vi "Main.vi"() -> ()   [LabVIEW 2013]
doc: "Use this template to build a simple state machine design pattern. Each state executes code and determines which state to transition to."
uses:
  controls/State.ctl
  controls/Data.ctl
panel:
  out "concatenated string":string
  out "Time to be saved":string
  out "String to be saved":string
  out "refnum out":refnum<file>
  in  "Feeder Input":i16=1
  in  "Corridor Input":i16=2
  in  "Feeder Delay":u32=500
  in  "Corridor Delay":u32=500
  in  "Sample Delay":i32=50
  out "Beam":u32
  in  "@Feeder":bool
  in  "Feeder Enable":bool
  in  "EoCo":bool
  in  "Exit":bool
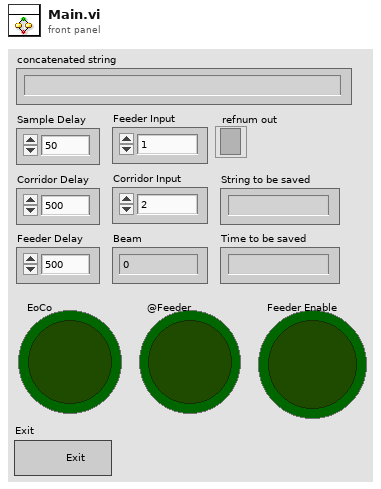
[diagram p1: front panel]
types:
  T1 = typedef "Data.ctl" = cluster{"String <Replace Me>":string, "Time Stamp":timestamp}
  T2 = typedef "State.ctl" = enum16{"Initialize", "Refresh", "Wait for Event", "End of Corridor", "End of Corridor Delay", "Feed", "Feed Delay", "Exit"}
  T3 = enum16{"open", "replace", "create", "open or create", "replace or create", "replace or create with confirmation"}
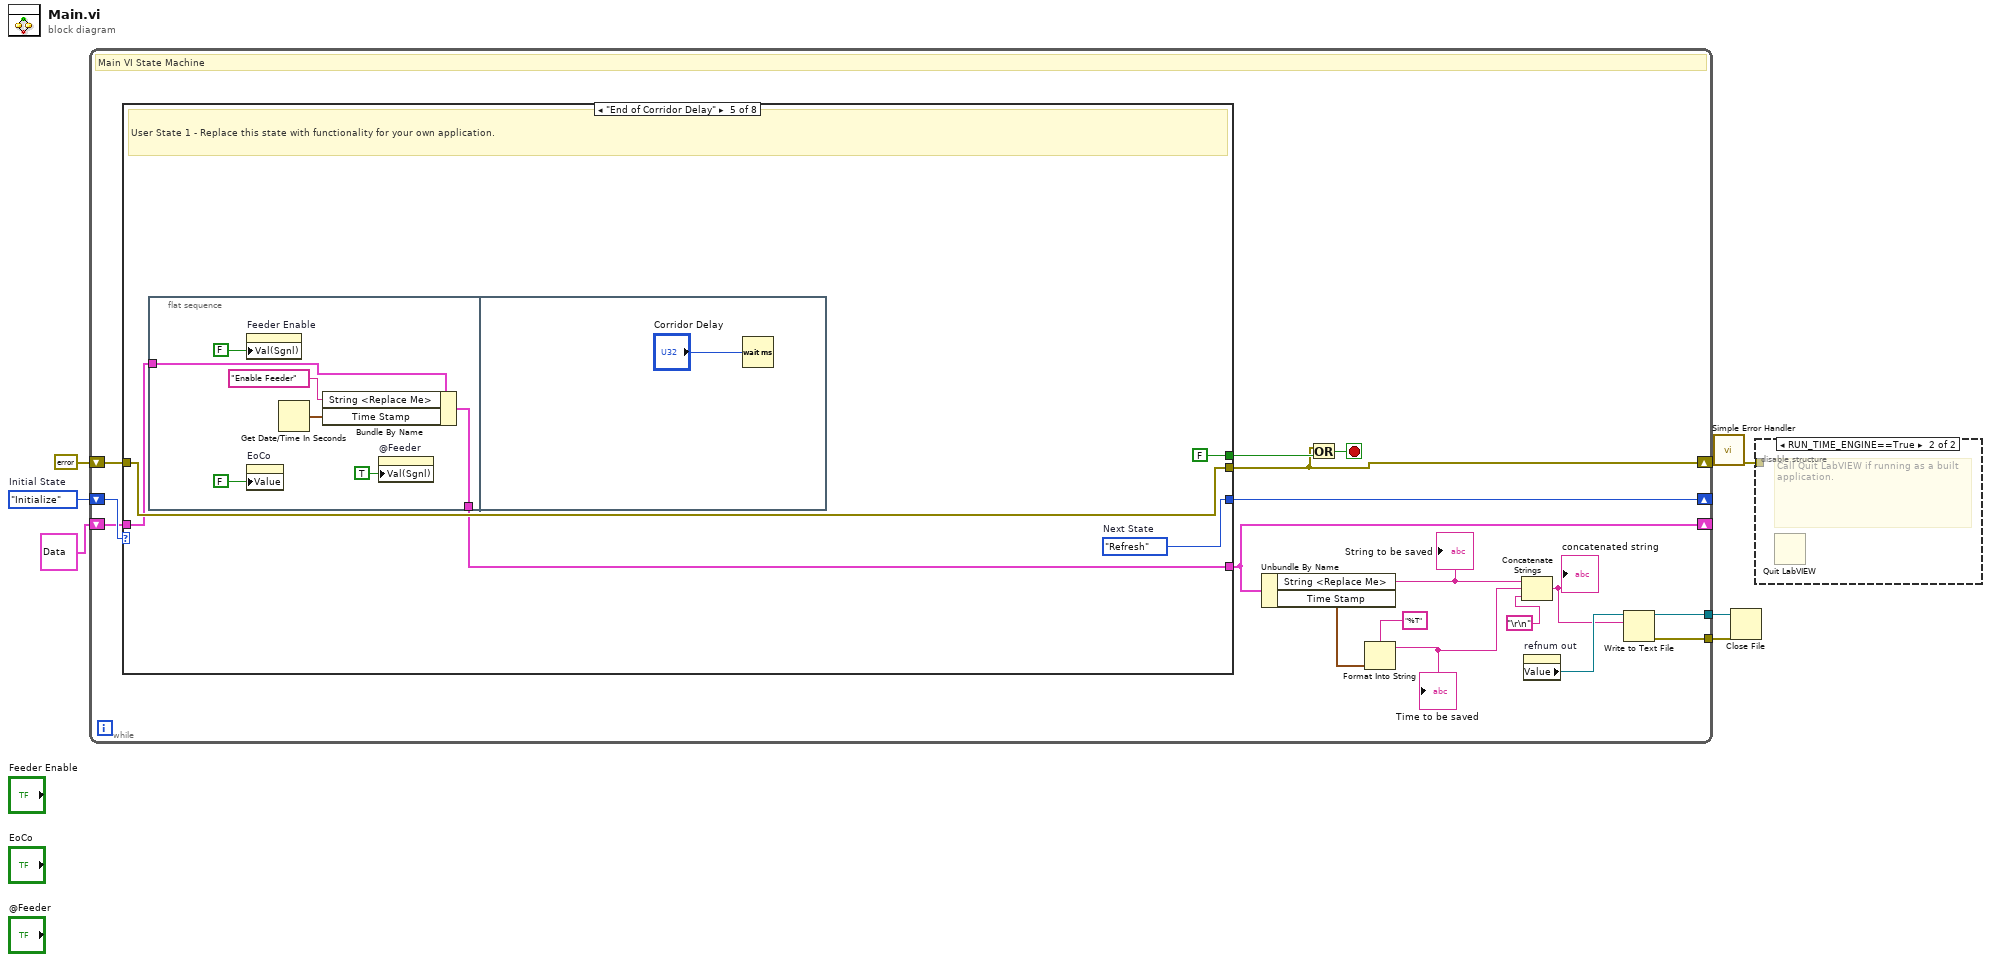
[diagram p0: block diagram]
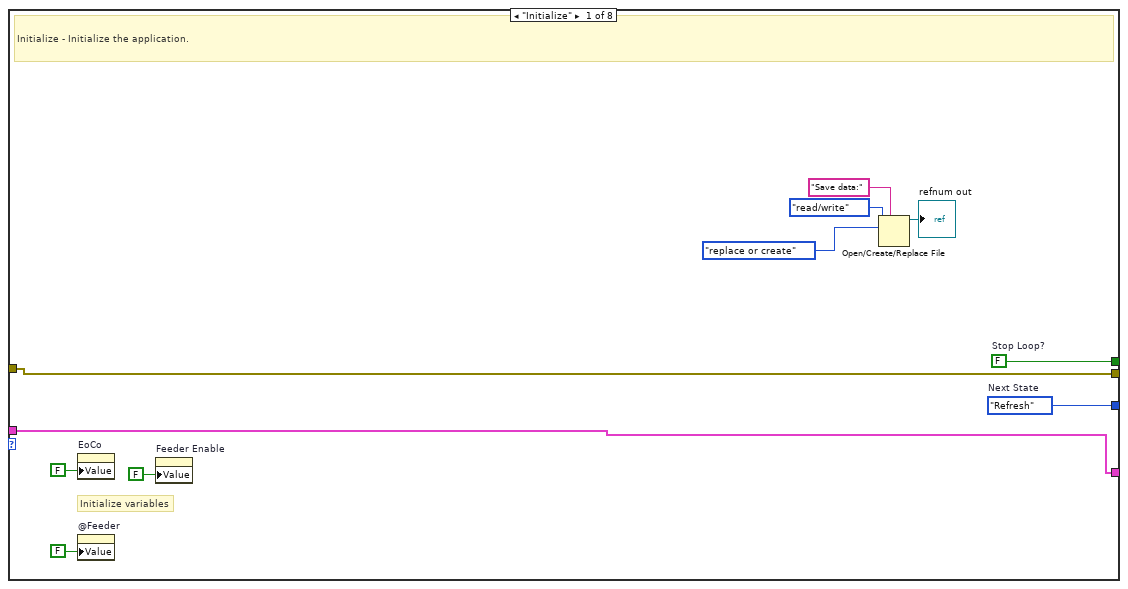
[diagram p3: hidden frame]
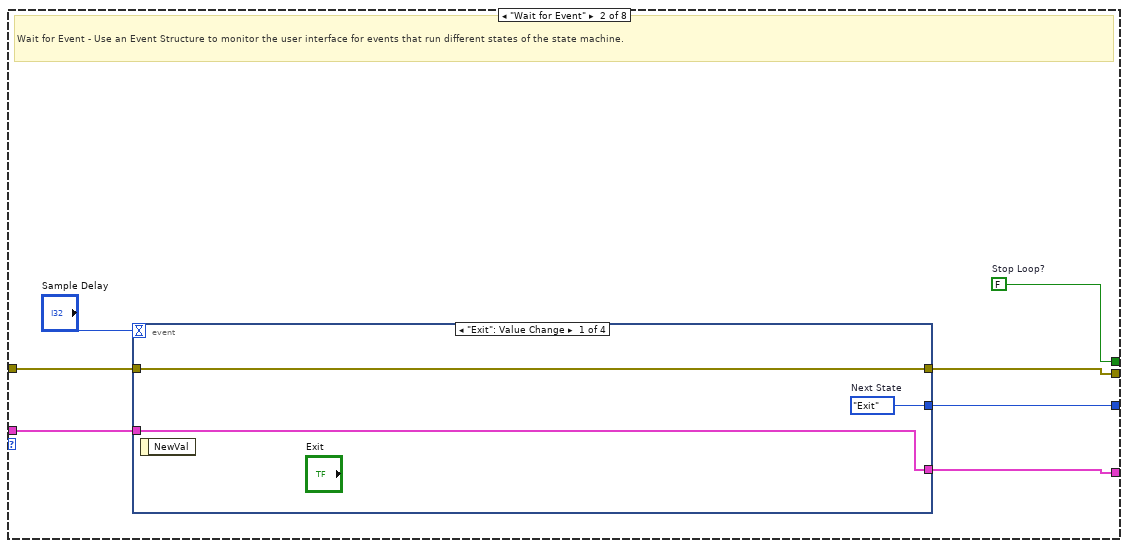
[diagram p4: hidden frame]
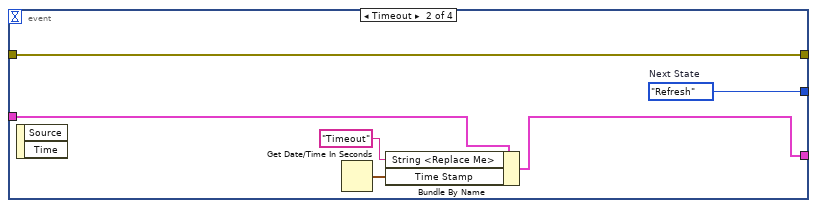
[diagram p5: hidden frame]
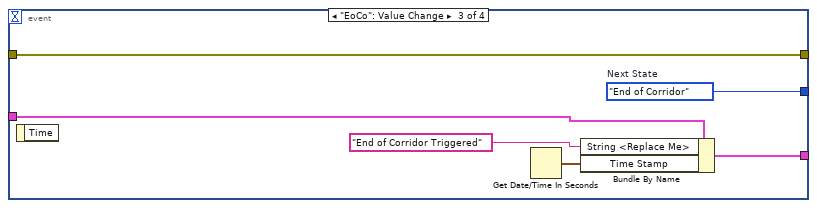
[diagram p6: hidden frame]
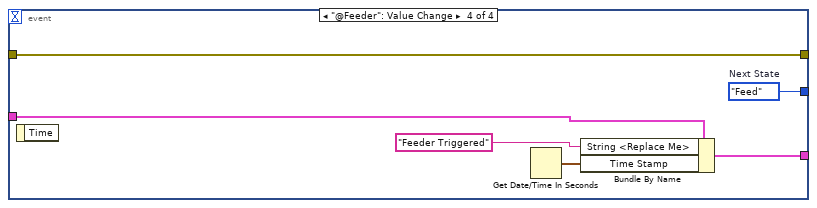
[diagram p7: hidden frame]
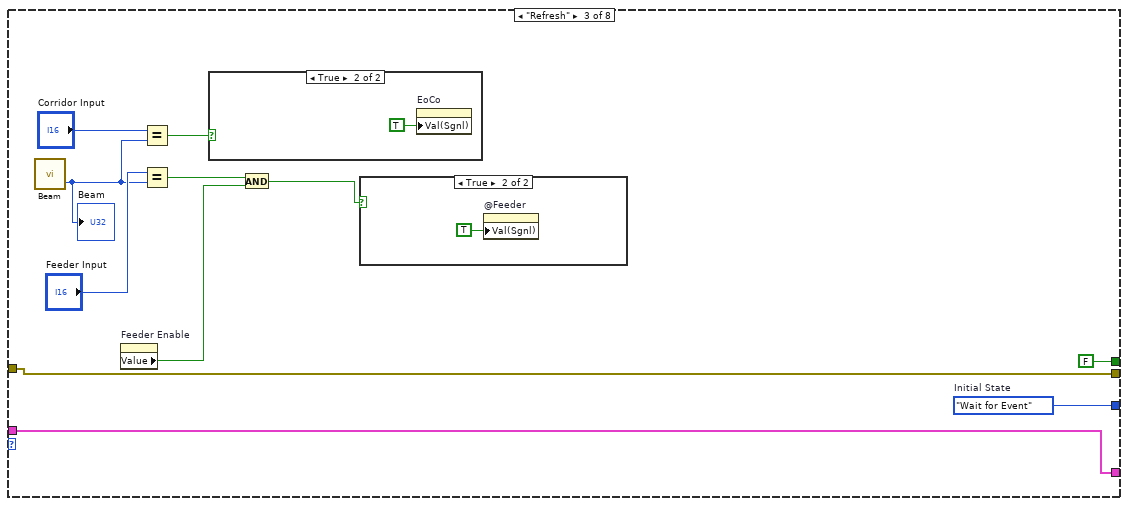
[diagram p8: hidden frame]
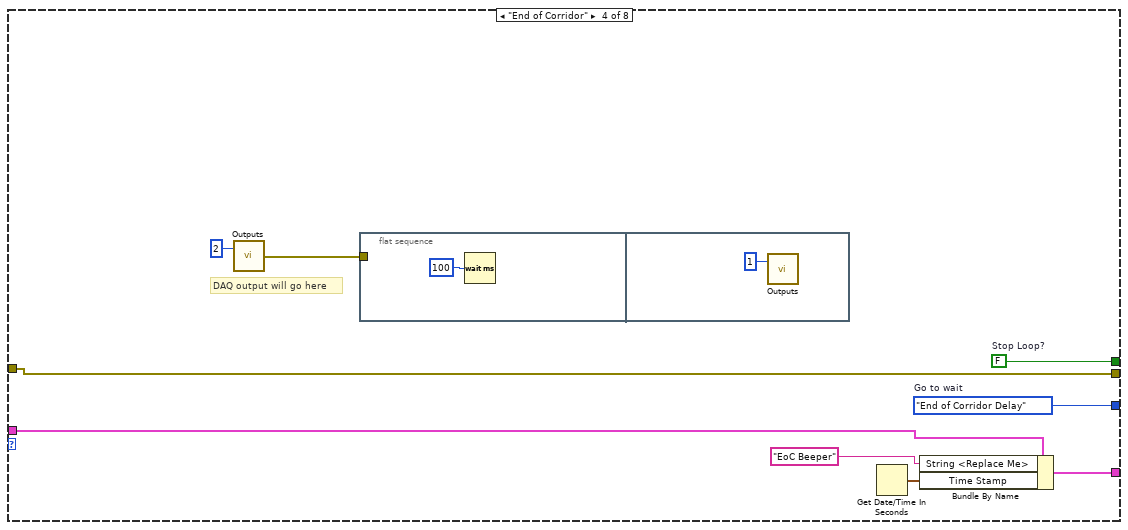
[diagram p11: hidden frame]
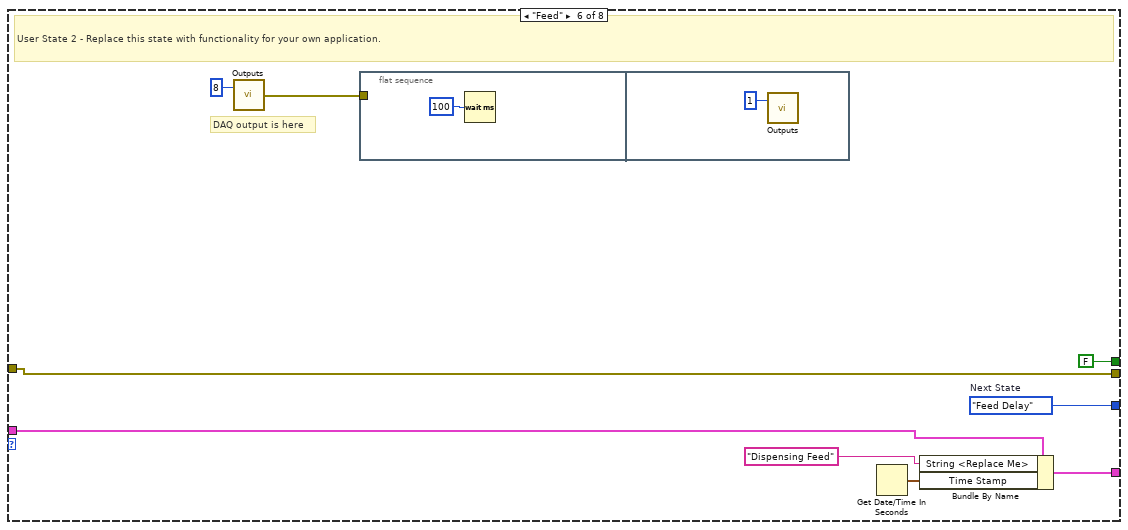
[diagram p12: hidden frame]
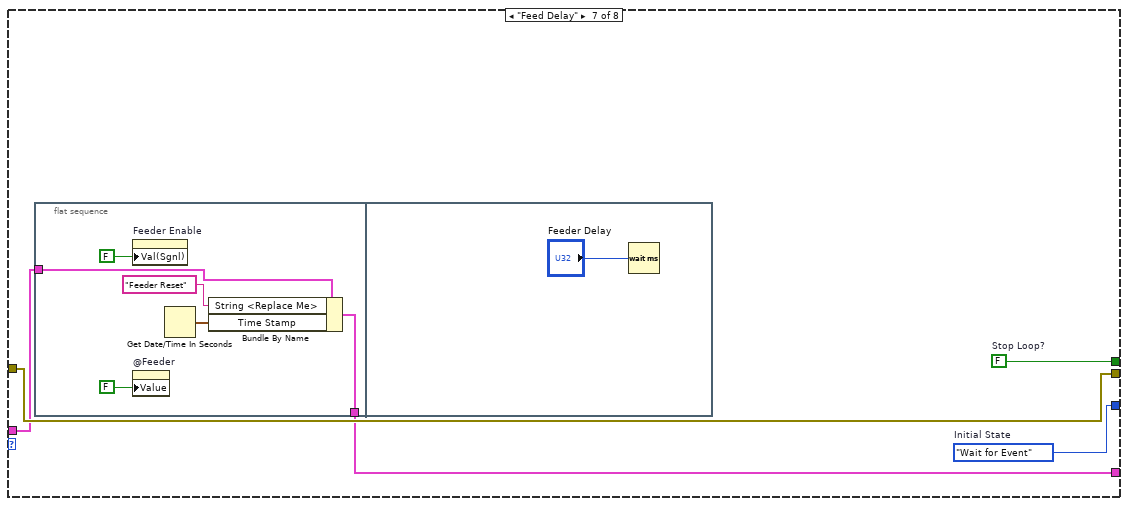
[diagram p13: hidden frame]
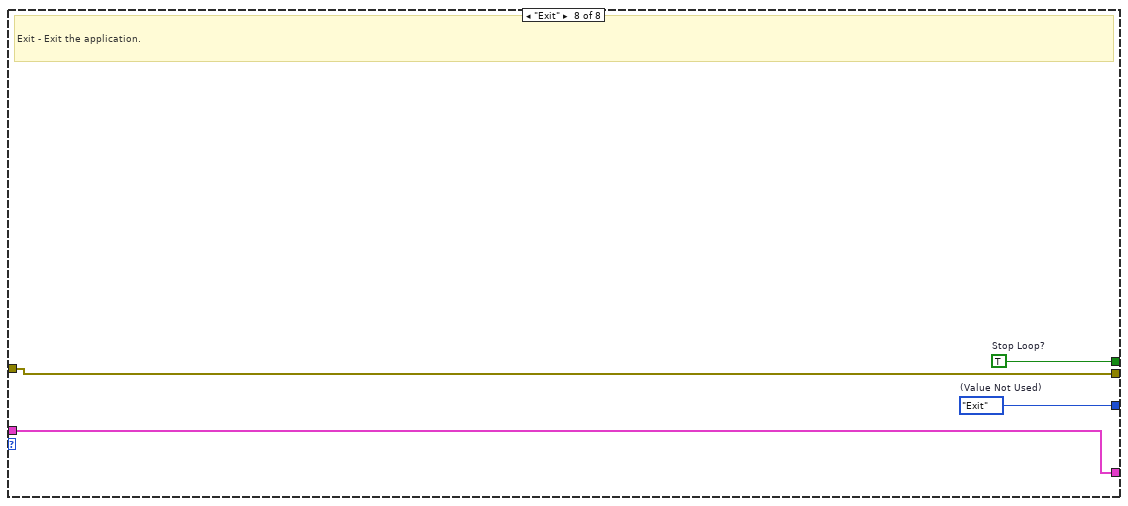
[diagram p14: hidden frame]
diagram:
  w7 = State."Initialize"  # Initial State
  n1 = while {
    shift-right: [w23] -> _
    shift-left: w7 -> [w24]
    shift-right: [w17] -> _
    shift-left: T1 {"String <Replace Me>"="", "Time Stamp"=timestamp(0 s since 1904-01-01)} ("Data") -> [w22]
    shift-right: [w18] -> w4
    shift-left: errorcluster {"status"=FALSE, "code"=0, "source"=""} ("error constant") -> [w21]
    tunnel: [w10] -> w2
    tunnel: [w9] -> w1
    stop <- w19 stop-if-true
    # "Main VI State Machine"
    n2 = case shown="\"End of Corridor Delay\"" w24 {
      tunnel: [w35 w42 w72 w84 w92 w109 w115 w127] -> w23
      tunnel: [w34 w41 FALSE ("Stop Loop?") w83 FALSE ("Stop Loop?") FALSE ("Stop Loop?") w114 w124] -> w20
      tunnel: w22 -> [w29 w40 w74 w78 w89 w104 w113 w126]
      tunnel: [w29 w39 w74 w77 w88 w103 w112 w126] -> w17
      tunnel: w21 -> [w33 w38 w73 w85 w90 w107 w116 w125]
      tunnel: [w33 w37 w73 w85 w90 w107 w116 w125] -> w18
      frame "Initialize" {
        w34 = FALSE  # Stop Loop?
        w35 = State."Refresh"  # Next State
        # "Initialize variables"
        # "Initialize - Initialize the application."
        n3 = property on="EoCo" class="Bool (strict)"("Value"=FALSE ("Value (Signaling)")) -> ()  [unwired: 2 in, 2 out]
        n4 = property on="@Feeder" class="Bool (strict)"("Value"=FALSE ("@Feeder")) -> ()  [unwired: 2 in, 2 out]
        n5 = property on="Feeder Enable" class="Bool (strict)"("Value"=FALSE) -> ()  [unwired: 2 in, 2 out]
        n6 = Open/Create/Replace File(prompt="Save data:", operation (0:open)=T3."replace or create", access (0:read/write)=enum16{"read/write", "read-only", "write-only"}."read/write") -> (refnum out=→"refnum out":refnum<file>)  [unwired: 3 in, 2 out]
      }
      frame "Wait for Event" {
        w41 = FALSE  # Stop Loop?
        # "Wait for Event - Use an Event Structure to monitor the user interface for events that run different states of the state machine."
        n7 = event shown="[0] \"Exit\": Value Change" {
          selector: _ -> [_ _ _ _]
          dyn-events: _ -> [_ _ _ _]
          timeout: "Sample Delay" -> [_ _ _ _]
          tunnel: [w45 w50 w57 w63] -> w42
          tunnel: w40 -> [w44 w48 w56 w62]
          tunnel: [w44 w47 w55 w61] -> w39
          tunnel: w38 -> [w43 w51 w53 w59]
          tunnel: [w43 w51 w53 w59] -> w37
          event "Exit": Value Change {
            w45 = State."Exit"  # Next State
            n8 = event-data() -> ()  [unwired: 1 in, 1 out]
          }
          event Timeout {
            w50 = State."Refresh"  # Next State
            n9 = event-data() -> ()  [unwired: 1 in, 2 out]
            n10 = Get Date/Time In Seconds() -> (seconds since 1Jan1904=w49:timestamp)
            n11 = Bundle By Name(cluster=w48, "String <Replace Me>"="Timeout", "Time Stamp"=w49) -> (w47:T1)
          }
          event "EoCo": Value Change {
            w57 = State."End of Corridor"  # Next State
            n12 = event-data() -> ()  [unwired: 1 in, 1 out]
            n13 = Get Date/Time In Seconds() -> (seconds since 1Jan1904=w52:timestamp)
            n14 = Bundle By Name(cluster=w56, "String <Replace Me>"="End of Corridor Triggered" ("Running User State 1"), "Time Stamp"=w52) -> (w55:T1)
          }
          event "@Feeder": Value Change {
            w63 = State."Feed"  # Next State
            n15 = event-data() -> ()  [unwired: 1 in, 1 out]
            n16 = Get Date/Time In Seconds() -> (seconds since 1Jan1904=w58:timestamp)
            n17 = Bundle By Name(cluster=w62, "String <Replace Me>"="Feeder Triggered" ("Running User State 2"), "Time Stamp"=w58) -> (w61:T1)
          }
        }
      }
      frame "Refresh" {
        w72 = State."Wait for Event"  # Initial State
        n18 = call "Beam.vi"() -> ("return type"=w64:i16)  [unwired: 1 in, 1 out]
        "Beam" <- w64
        n19 = property on="Feeder Enable" class="Bool (strict)"() -> ("Value"=w71:bool)  [unwired: 2 in, 2 out]
        n20 = Equal?(x="Corridor Input", y=w64) -> (x = y?=w68:bool)
        n21 = Equal?(x="Feeder Input", y=w64) -> (x = y?=w69:bool)
        n22 = case shown="True" w68 {
          frame False {
          }
          frame True {
            n23 = property on="EoCo" class="Bool (strict)"("Val(Sgnl)"=TRUE ("Value (Signaling)")) -> ()  [unwired: 2 in, 2 out]
          }
        }
        n24 = And(x=w69, y=w71) -> (x .and. y?=w70:bool)
        n25 = case shown="True" w70 {
          frame False {
          }
          frame True {
            n26 = property on="@Feeder" class="Bool (strict)"("Val(Sgnl)"=TRUE ("Value (Signaling)")) -> ()  [unwired: 2 in, 2 out]
          }
        }
      }
      frame "End of Corridor" {
        w83 = FALSE  # Stop Loop?
        w84 = State."End of Corridor Delay"  # Go to wait
        # "DAQ output will go here"
        n27 = call "Outputs.vi"("Value"=i16 2) -> ("error out"=w82:errorcluster)  [unwired: 1 in]
        n28 = flat-sequence {
          tunnel: w82 -> [_]
          frame #0 {
            n29 = Wait (ms)(milliseconds to wait=u32 100) -> ()  [unwired: 1 out]
          }
          frame #1 {
            n30 = call "Outputs.vi"("Value"=i16 1) -> ()  [unwired: 1 in, 1 out]
          }
        }
        n31 = Get Date/Time In Seconds() -> (seconds since 1Jan1904=w79:timestamp)
        n32 = Bundle By Name(cluster=w78, "String <Replace Me>"="EoC Beeper", "Time Stamp"=w79) -> (w77:T1)
      }
      frame "End of Corridor Delay" {
        w92 = State."Refresh"  # Next State
        # "User State 1 - Replace this state with functionality for your own application."
        n33 = flat-sequence {
          tunnel: w89 -> [w95]
          tunnel: [w94] -> w88
          frame #0 {
            n34 = property on="Feeder Enable" class="Bool (strict)"("Val(Sgnl)"=FALSE ("Value (Signaling)")) -> ()  [unwired: 2 in, 2 out]
            n35 = property on="EoCo" class="Bool (strict)"("Value"=FALSE ("Value (Signaling)")) -> ()  [unwired: 2 in, 2 out]
            n36 = Get Date/Time In Seconds() -> (seconds since 1Jan1904=w97:timestamp)
            n37 = Bundle By Name(cluster=w95, "String <Replace Me>"="Enable Feeder", "Time Stamp"=w97) -> (w94:T1)
            n38 = property on="@Feeder" class="Bool (strict)"("Val(Sgnl)"=TRUE ("Value (Signaling)")) -> ()  [unwired: 2 in, 2 out]
          }
          frame #1 {
            n39 = Wait (ms)(milliseconds to wait="Corridor Delay") -> ()  [unwired: 1 out]
          }
        }
      }
      frame "Feed" {
        w109 = State."Feed Delay"  # Next State
        # "DAQ output is here"
        # "User State 2 - Replace this state with functionality for your own application."
        n40 = call "Outputs.vi"("Value"=i16 8) -> ("error out"=w106:errorcluster)  [unwired: 1 in]
        n41 = flat-sequence {
          tunnel: w106 -> [_]
          frame #0 {
            n42 = Wait (ms)(milliseconds to wait=u32 100) -> ()  [unwired: 1 out]
          }
          frame #1 {
            n43 = call "Outputs.vi"("Value"=i16 1) -> ()  [unwired: 1 in, 1 out]
          }
        }
        n44 = Get Date/Time In Seconds() -> (seconds since 1Jan1904=w102:timestamp)
        n45 = Bundle By Name(cluster=w104, "String <Replace Me>"="Dispensing Feed", "Time Stamp"=w102) -> (w103:T1)
      }
      frame "Feed Delay" {
        w114 = FALSE  # Stop Loop?
        w115 = State."Wait for Event"  # Initial State
        n46 = flat-sequence {
          tunnel: w113 -> [w118]
          tunnel: [w117] -> w112
          frame #0 {
            n47 = property on="Feeder Enable" class="Bool (strict)"("Val(Sgnl)"=FALSE ("Value (Signaling)")) -> ()  [unwired: 2 in, 2 out]
            n48 = property on="@Feeder" class="Bool (strict)"("Value"=FALSE ("@Feeder")) -> ()  [unwired: 2 in, 2 out]
            n49 = Get Date/Time In Seconds() -> (seconds since 1Jan1904=w119:timestamp)
            n50 = Bundle By Name(cluster=w118, "String <Replace Me>"="Feeder Reset", "Time Stamp"=w119) -> (w117:T1)
          }
          frame #1 {
            n51 = Wait (ms)(milliseconds to wait="Feeder Delay") -> ()  [unwired: 1 out]
          }
        }
      }
      frame "Exit" {
        w124 = TRUE  # Stop Loop?
        w127 = State."Exit"  # (Value Not Used)
        # "Exit - Exit the application."
      }
    }
    n52 = Unbundle By Name(w17) -> ("String <Replace Me>"=w13:string, "Time Stamp"=w16:timestamp)
    "String to be saved" <- w13
    n53 = Or(x=w18, y=w20) -> (x .or. y?=w19:bool)
    n54 = Format Into String(format string="%T", w16) -> (resulting string=w12:string)  [unwired: 2 in, 1 out]
    "Time to be saved" <- w12
    n55 = Concatenate Strings(w13, w12, "\r\n") -> (w11:string)
    "concatenated string" <- w11
    n56 = property on="refnum out" class="Ref (strict)"() -> ("Value"=w14:refnum<file>)  [unwired: 2 in, 2 out]
    n57 = Write to Text File(file (use dialog)=w14, text=w11) -> (refnum out=w9:refnum<file>, error out=w10:errorcluster)  [unwired: 2 in, 1 out]
  }
  n58 = call <vilib>:"Simple Error Handler.vi"("error in (no error)"=w4) -> ("error out"=w3:errorcluster)  [unwired: 4 in, 4 out]
  n59 = Close File(refnum=w1, error in=w2) -> ()  [unwired: 2 out]
  n60 = disable-structure shown="RUN_TIME_ENGINE==True" {
    disable-tunnel: w3 -> [_ _]
    frame condition #0 (active) {
    }
    frame condition #1 {
      # "Call Quit LabVIEW if running as a built application."
      n61 = Quit LabVIEW() -> ()  [unwired: 1 in]
    }
  }
